vi "SP_OEE_2_test.vi"() -> ()   [LabVIEW 2017] (continued)
                          disable-tunnel: w4489 -> [w4505 w4508]
                          disable-tunnel: [w4504 w4508] -> w4488
                          disable-tunnel: [w4503 w4509] -> w4487
                          disable-tunnel: w4486 -> [w4502 _]
                          disable-tunnel: w4485 -> [w4501 _]
                          disable-tunnel: [w4500 _] -> w4484
                          disable-tunnel: [w4499 _] -> w4480
                          disable-tunnel: w4478 -> [w4498 _]
                          frame Disabled {
                            n825 = call "Stack_holderwise_total_bd_count_&_duration.vi"("Refnum in"=w4505, "BREAKDOWN_STK_HOLD_ID"=4, "condition"=w4498, "Form Date"=w4502, "To Date"=w4501, "error in (no error)"=w4506) -> ("Refnum out"=w4504:T2, "Count out"=w4500:string[], "appended array"=w4499:dbl[], "error out"=w4503:errorcluster)  [unwired: 6 in]
                          }
                          frame Enabled {
                          }
                        }
                        n826 = call "Insert_empty_element_with_zero.vi"("searched date"=w4484, "fixed date"=w4481) -> ("O/P"=w4483:string[])  [unwired: 9 in]
                        n827 = call "NUMERIC TO STRING.vi"("appended array"=w4480) -> ("Array"=w4479:string[])  [unwired: 4 in]
                        n828 = call "Insert_empty_element_with_zero.vi"("searched date"=w4479, "fixed date"=w4481) -> ("O/P"=w4482:string[])  [unwired: 9 in]
                      }
                      frame #5 {
                        n829 = disable-structure shown="Enabled" {
                          disable-tunnel: w4523 -> [w4541 w4544]
                          disable-tunnel: [w4540 w4544] -> w4522
                          disable-tunnel: w4521 -> [w4539 w4543]
                          disable-tunnel: [w4538 w4543] -> w4520
                          disable-tunnel: w4519 -> [w4537 _]
                          disable-tunnel: w4518 -> [w4536 _]
                          disable-tunnel: [w4535 _] -> w4517
                          disable-tunnel: [w4534 _] -> w4513
                          disable-tunnel: w4511 -> [w4533 _]
                          frame Disabled {
                            n830 = call "Stack_holderwise_total_bd_count_&_duration.vi"("Refnum in"=w4539, "BREAKDOWN_STK_HOLD_ID"=5, "condition"=w4533, "Form Date"=w4536, "To Date"=w4537, "error in (no error)"=w4541) -> ("Refnum out"=w4538:T2, "Count out"=w4535:string[], "appended array"=w4534:dbl[], "error out"=w4540:errorcluster)  [unwired: 6 in]
                          }
                          frame Enabled {
                          }
                        }
                        n831 = call "NUMERIC TO STRING.vi"("appended array"=w4513) -> ("Array"=w4512:string[])  [unwired: 4 in]
                        n832 = call "Insert_empty_element_with_zero.vi"("searched date"=w4517, "fixed date"=w4515) -> ("O/P"=w4516:string[])  [unwired: 9 in]
                        n833 = call "Insert_empty_element_with_zero.vi"("searched date"=w4512, "fixed date"=w4515) -> ("O/P"=w4514:string[])  [unwired: 9 in]
                      }
                      frame #6 {
                        n834 = call "String to numeric.vi"("Array"=w4555) -> ("Array 2"=w4554:dbl[])  [unwired: 4 in]
                        n835 = call "String to numeric.vi"("Array"=w4553) -> ("Array 2"=w4552:dbl[])  [unwired: 4 in]
                        n836 = call "String to numeric.vi"("Array"=w4551) -> ("Array 2"=w4550:dbl[])  [unwired: 4 in]
                        n837 = call "String to numeric.vi"("Array"=w4549) -> ("Array 2"=w4548:dbl[])  [unwired: 4 in]
                        n838 = call "String to numeric.vi"("Array"=w4547) -> ("Array 2"=w4546:dbl[])  [unwired: 4 in]
                        n839 = Decimal String To Number(string=w4560) -> (number=w4579:i32[])  [unwired: 2 in, 1 out]
                        n840 = Decimal String To Number(string=w4561) -> (number=w4580:i32[])  [unwired: 2 in, 1 out]
                        n841 = Decimal String To Number(string=w4562) -> (number=w4581:i32[])  [unwired: 2 in, 1 out]
                        n842 = Decimal String To Number(string=w4563) -> (number=w4582:i32[])  [unwired: 2 in, 1 out]
                        n843 = Decimal String To Number(string=w4564) -> (number=w4577:i32[])  [unwired: 2 in, 1 out]
                        n844 = Compound Arithmetic op=ADD(w4554, w4552, w4550, w4548, w4546) -> (w4557:dbl[])
                        n845 = Build Array(w4555) -> (w4576:string[][])
                        n846 = Build Array(w4553) -> (w4575:string[][])
                        n847 = Build Array(w4551) -> (w4574:string[][])
                        n848 = Build Array(w4549) -> (w4573:string[][])
                        n849 = Build Array(w4547) -> (w4572:string[][])
                        n850 = Number To Fractional String(number=w4557, precision (6)=i16 2) -> (F-format string=w4556:string[])  [unwired: 2 in]
                        n851 = Compound Arithmetic op=ADD(w4579, w4580, w4581, w4582, w4577) -> (w4583:i32[])
                        n852 = Transpose 2D Array(2D array=w4576) -> (transposed array=w4570:string[][])
                        n853 = Transpose 2D Array(2D array=w4575) -> (transposed array=w4569:string[][])
                        n854 = Transpose 2D Array(2D array=w4574) -> (transposed array=w4568:string[][])
                        n855 = Transpose 2D Array(2D array=w4573) -> (transposed array=w4567:string[][])
                        n856 = Transpose 2D Array(2D array=w4572) -> (transposed array=w4566:string[][])
                        n857 = Number To Decimal String(number=w4583) -> (decimal integer string=w4578:string[])  [unwired: 1 in]
                        n858 = Build Array(w4556) -> (w4559:string[][])
                        n859 = Transpose 2D Array(2D array=w4559) -> (transposed array=w4565:string[][])
                      }
                      frame #7 {
                        w4587 = string[] [""]
                        n860 = Insert Into Array(array=w4597, index (col)=1 ("disabled index (col)"), new element #1=w4587, new element #2=w4587, new element #3=w4588, new element #4=w4589, new element #5=w4587, new element #6=w4587, new element #7=w4587, new element #8=w4587, new element #9=w4587, new element #10=w4587, new element #11=w4590, new element #12=w4591) -> (w4593:string[][])  [unwired: 1 in]
                        n861 = call "flot graph for month n year.vi"("BD Date"=w4594, "error in (no error)"=w4596, "Count total"=w4590) -> ("error out"=w4595:errorcluster, "Run-Time Status"=w4592:cluster{"Array 2":timestamp[], dbl[]})  [unwired: 7 in]
                        n862 = local write "Run-Time Status"(w4592) -> ()
                        n863 = local write "Table"(w4593) -> ()
                      }
                    }
                  }
                  frame "all" {
                  }
                }
              }
              frame "Maintenance" {
                n864 = local read "Shift"() -> (w4599:string)
                n865 = case shown="\"1\"" w4599 {
                  selector: w4599 -> [_ w4972 w5351 w5730 _]
                  tunnel: w4604 -> [w4609 w4977 w5356 w5735 _]
                  tunnel: w4603 -> [w4608 w4976 w5355 w5734 _]
                  tunnel: w4602 -> [w4607 w4975 w5354 w5733 _]
                  tunnel: w4601 -> [w4606 w4974 w5353 w5732 _]
                  tunnel: w4600 -> [w4605 w4973 w5352 w5731 _]
                  frame "ALL", Default {
                    n866 = flat-sequence {
                      tunnel: w4609 -> [w4721]
                      tunnel: w4608 -> [w4719]
                      tunnel: [w4705] -> w4699
                      tunnel: [w4720] -> w4698
                      tunnel: w4607 -> [_]
                      tunnel: [w4724] -> w4697
                      tunnel: [w4704] -> w4696
                      tunnel: [w4703] -> w4695
                      tunnel: [w4701] -> w4694
                      tunnel: w4606 -> [w4704]
                      tunnel: w4605 -> [w4703]
                      tunnel: ["Where BREAKDOWN_DATE between '%s'and '%s' and BREAKDOWN_STK_HOLD_ID ='%d'  "] -> w4693
                      tunnel: [w4701] -> w4692
                      tunnel: w4699 -> [w4783]
                      tunnel: w4698 -> [w4785]
                      tunnel: w4697 -> [w4781]
                      tunnel: w4696 -> [w4780]
                      tunnel: w4695 -> [w4779]
                      tunnel: [w4782] -> w4691
                      tunnel: [w4784] -> w4690
                      tunnel: [w4781] -> w4689
                      tunnel: [w4771] -> w4688
                      tunnel: [w4777] -> w4687
                      tunnel: [w4780] -> w4686
                      tunnel: [w4779] -> w4685
                      tunnel: w4694 -> [w4776]
                      tunnel: [w4776] -> w4684
                      tunnel: w4693 -> [w4773]
                      tunnel: [w4773] -> w4683
                      tunnel: [w4772] -> w4682
                      tunnel: w4692 -> [w4772]
                      tunnel: w4691 -> [w4811]
                      tunnel: w4690 -> [w4809]
                      tunnel: w4689 -> [w4814]
                      tunnel: w4688 -> [w4813]
                      tunnel: w4687 -> [w4812]
                      tunnel: w4686 -> [w4807]
                      tunnel: w4685 -> [w4806]
                      tunnel: [w4814] -> w4681
                      tunnel: [w4813] -> w4680
                      tunnel: [w4812] -> w4679
                      tunnel: [w4810] -> w4678
                      tunnel: [w4804] -> w4677
                      tunnel: [w4803] -> w4676
                      tunnel: [w4808] -> w4675
                      tunnel: [w4807] -> w4674
                      tunnel: [w4806] -> w4673
                      tunnel: w4684 -> [w4802]
                      tunnel: [w4802] -> w4672
                      tunnel: w4683 -> [w4799]
                      tunnel: [w4799] -> w4671
                      tunnel: [w4798] -> w4670
                      tunnel: w4682 -> [w4798]
                      tunnel: w4681 -> [w4846]
                      tunnel: w4680 -> [w4845]
                      tunnel: w4679 -> [w4844]
                      tunnel: w4678 -> [w4841]
                      tunnel: w4677 -> [w4843]
                      tunnel: w4676 -> [w4842]
                      tunnel: w4675 -> [w4839]
                      tunnel: w4674 -> [w4837]
                      tunnel: w4673 -> [w4836]
                      tunnel: [w4846] -> w4669
                      tunnel: [w4845] -> w4668
                      tunnel: [w4844] -> w4667
                      tunnel: [w4843] -> w4666
                      tunnel: [w4842] -> w4665
                      tunnel: [w4840] -> w4664
                      tunnel: [w4834] -> w4663
                      tunnel: [w4833] -> w4662
                      tunnel: [w4838] -> w4661
                      tunnel: [w4837] -> w4660
                      tunnel: [w4836] -> w4659
                      tunnel: w4672 -> [w4832]
                      tunnel: [w4832] -> w4658
                      tunnel: w4671 -> [w4829]
                      tunnel: [w4829] -> w4657
                      tunnel: [w4828] -> w4656
                      tunnel: w4670 -> [w4828]
                      tunnel: w4669 -> [w4867]
                      tunnel: w4668 -> [w4866]
                      tunnel: w4667 -> [w4865]
                      tunnel: w4666 -> [w4864]
                      tunnel: w4665 -> [w4863]
                      tunnel: w4664 -> [w4860]
                      tunnel: w4663 -> [w4862]
                      tunnel: w4662 -> [w4861]
                      tunnel: w4661 -> [w4859]
                      tunnel: w4660 -> [w4856]
                      tunnel: w4659 -> [w4855]
                      tunnel: [w4867] -> w4655
                      tunnel: [w4866] -> w4654
                      tunnel: [w4865] -> w4653
                      tunnel: [w4864] -> w4652
                      tunnel: [w4863] -> w4651
                      tunnel: [w4862] -> w4650
                      tunnel: [w4861] -> w4649
                      tunnel: [w4858] -> w4648
                      tunnel: [w4857] -> w4647
                      tunnel: [w4853] -> w4646
                      tunnel: [w4852] -> w4645
                      tunnel: [w4856] -> w4644
                      tunnel: [w4855] -> w4643
                      tunnel: w4658 -> [w4851]
                      tunnel: [w4851] -> w4642
                      tunnel: w4657 -> [w4848]
                      tunnel: [w4848] -> w4641
                      tunnel: [w4847] -> w4640
                      tunnel: w4656 -> [w4847]
                      tunnel: w4655 -> [w4902]
                      tunnel: w4654 -> [w4901]
                      tunnel: w4653 -> [w4900]
                      tunnel: w4652 -> [w4899]
                      tunnel: w4651 -> [w4898]
                      tunnel: w4650 -> [w4897]
                      tunnel: w4649 -> [w4896]
                      tunnel: w4648 -> [w4891]
                      tunnel: w4647 -> [w4893]
                      tunnel: w4646 -> [w4895]
                      tunnel: w4645 -> [w4894]
                      tunnel: w4644 -> [w4888]
                      tunnel: w4643 -> [w4889]
                      tunnel: [w4902] -> w4639
                      tunnel: [w4901] -> w4638
                      tunnel: [w4900] -> w4637
                      tunnel: [w4899] -> w4636
                      tunnel: [w4898] -> w4635
                      tunnel: [w4897] -> w4634
                      tunnel: [w4896] -> w4633
                      tunnel: [w4895] -> w4632
                      tunnel: [w4894] -> w4631
                      tunnel: [w4892] -> w4630
                      tunnel: [w4890] -> w4629
                      tunnel: [w4886] -> w4628
                      tunnel: [w4884] -> w4627
                      tunnel: w4642 -> [w4885]
                      tunnel: w4641 -> [w4881]
                      tunnel: [w4880] -> w4626
                      tunnel: w4640 -> [w4880]
                      tunnel: w4639 -> [w4941]
                      tunnel: w4638 -> [w4934]
                      tunnel: w4637 -> [w4925]
                      tunnel: w4636 -> [w4933]
                      tunnel: w4635 -> [w4923]
                      tunnel: w4634 -> [w4932]
                      tunnel: w4633 -> [w4921]
                      tunnel: w4632 -> [w4931]
                      tunnel: w4631 -> [w4919]
                      tunnel: w4630 -> [w4955]
                      tunnel: w4629 -> [w4954]
                      tunnel: w4628 -> [w4930]
                      tunnel: w4627 -> [w4917]
                      tunnel: [w4955] -> w4625
                      tunnel: [w4954] -> w4624
                      tunnel: [w4948] -> w4623
                      tunnel: [w4941] -> w4622
                      tunnel: [w4940] -> w4621
                      tunnel: [w4939] -> w4620
                      tunnel: [w4938] -> w4619
                      tunnel: [w4937] -> w4618
                      tunnel: [w4936] -> w4617
                      tunnel: [w4935] -> w4616
                      tunnel: [w4934] -> w4615
                      tunnel: [w4933] -> w4614
                      tunnel: [w4932] -> w4613
                      tunnel: [w4931] -> w4612
                      tunnel: [w4930] -> w4611
                      tunnel: [w4915] -> w4610
                      tunnel: w4626 -> [w4915]
                      tunnel: [w4968] -> _
                      tunnel: [w4964] -> _
                      tunnel: w4625 -> [w4965]
                      tunnel: w4624 -> [w4968]
                      tunnel: w4623 -> [w4959]
                      tunnel: w4622 -> [w4966]
                      tunnel: w4621 -> [_]
                      tunnel: w4620 -> [_]
                      tunnel: w4619 -> [w4956]
                      tunnel: w4618 -> [_]
                      tunnel: w4617 -> [_]
                      tunnel: w4616 -> [w4960]
                      tunnel: w4615 -> [_]
                      tunnel: w4614 -> [_]
                      tunnel: w4613 -> [w4957]
                      tunnel: w4612 -> [_]
                      tunnel: w4611 -> [_]
                      tunnel: w4610 -> [w4963]
                      frame #0 {
                        w4712 = "%Y-%m-%d" ("time format string (%c)")
                        n867 = property on="Table" class="Tbl (strict)"("Visible"=TRUE) -> ()  [unwired: 2 in, 2 out]
                        n868 = Format Date/Time String(time format string (%c)=w4712, seconds (now)=w4704) -> (date/time string=w4713:string)  [unwired: 1 in]
                        n869 = Format Date/Time String(time format string (%c)=w4712, seconds (now)=w4703) -> (date/time string=w4711:string)  [unwired: 1 in]
                        n870 = Format Into String(format string="Where BREAKDOWN_DATE between '%s' and '%s' ", w4713, w4711) -> (resulting string=w4710:string)  [unwired: 2 in, 1 out]
                        n871 = call <vilib>:"DB Tools Select Data.vi"("condition"=w4710, "error in (no error)"=w4719, "columns"=string[] ["BREAKDOWN_DATE"], "table"="STATION_1_LOG_HISTORY", "connection reference"=w4721) -> ("error out"=w4706:errorcluster, "data"=w4709:variant[][], "connection reference out"=w4720:T2)  [unwired: 1 in]
                        n872 = property on="Table 2" class="Tbl (strict)"("Visible"=FALSE) -> ()  [unwired: 2 in, 2 out]
                        n873 = xnode "Database Variant To Data"("database variant"=w4709, "error in (no error)"=w4706, "type"=string[][] [] ("Elements Found")) -> ("data"=w4707:string[][], "error out"=w4705:errorcluster)
                        n874 = Index Array(array=w4707, index (col)=0 ("disabled index (col)")) -> (element=w4715:string[])  [unwired: 1 in]
                        n875 = call "Search_1d_array_element.vi"("Count in"=string[] [] ("Elements Found"), "BD Date"=w4715, "Elements Found in"=string[] [] ("Elements Found")) -> ("Elements Found out"=w4701:string[])  [unwired: 4 in, 2 out]
                        n876 = Build Array(w4701) -> (w4725:string[][])
                        n877 = Transpose 2D Array(2D array=w4725) -> (transposed array=w4724:string[][])
                      }
                      frame #1 {
                        n878 = disable-structure shown="Enabled" {
                          disable-tunnel: w4785 -> [w4795 w4796]
                          disable-tunnel: [w4794 w4796] -> w4784
                          disable-tunnel: w4783 -> [w4793 w4797]
                          disable-tunnel: [w4792 w4797] -> w4782
                          disable-tunnel: w4780 -> [w4790 _]
                          disable-tunnel: w4779 -> [w4789 _]
                          disable-tunnel: [w4788 _] -> w4778
                          disable-tunnel: [w4787 _] -> w4775
                          disable-tunnel: w4773 -> [w4786 _]
                          frame Disabled {
                            n879 = call "Stack_holderwise_total_bd_count_&_duration.vi"("Refnum in"=w4795, "BREAKDOWN_STK_HOLD_ID"=1, "condition"=w4786, "Form Date"=w4790, "To Date"=w4789, "error in (no error)"=w4793) -> ("Refnum out"=w4794:T2, "Count out"=w4788:string[], "appended array"=w4787:dbl[], "error out"=w4792:errorcluster)  [unwired: 6 in]
                          }
                          frame Enabled {
                          }
                        }
                        n880 = call "NUMERIC TO STRING.vi"("appended array"=w4775) -> ("Array"=w4774:string[])  [unwired: 4 in]
                        n881 = call "Insert_empty_element_with_zero.vi"("searched date"=w4778, "fixed date"=w4776) -> ("O/P"=w4771:string[])  [unwired: 9 in]
                        n882 = call "Insert_empty_element_with_zero.vi"("searched date"=w4774, "fixed date"=w4776) -> ("O/P"=w4777:string[])  [unwired: 9 in]
                      }
                      frame #2 {
                        n883 = disable-structure shown="Enabled" {
                          disable-tunnel: w4811 -> [w4824 w4826]
                          disable-tunnel: [w4823 w4826] -> w4810
                          disable-tunnel: w4809 -> [w4822 w4825]
                          disable-tunnel: [w4821 w4825] -> w4808
                          disable-tunnel: w4807 -> [w4820 _]
                          disable-tunnel: w4806 -> [w4819 _]
                          disable-tunnel: [w4818 _] -> w4805
                          disable-tunnel: [w4817 _] -> w4801
                          disable-tunnel: w4799 -> [w4816 _]
                          frame Disabled {
                            n884 = call "Stack_holderwise_total_bd_count_&_duration.vi"("Refnum in"=w4822, "BREAKDOWN_STK_HOLD_ID"=2, "condition"=w4816, "Form Date"=w4820, "To Date"=w4819, "error in (no error)"=w4824) -> ("Refnum out"=w4821:T2, "Count out"=w4818:string[], "appended array"=w4817:dbl[], "error out"=w4823:errorcluster)  [unwired: 6 in]
                          }
                          frame Enabled {
                          }
                        }
                        n885 = call "Insert_empty_element_with_zero.vi"("searched date"=w4805, "fixed date"=w4802) -> ("O/P"=w4804:string[])  [unwired: 9 in]
                        n886 = call "NUMERIC TO STRING.vi"("appended array"=w4801) -> ("Array"=w4800:string[])  [unwired: 4 in]
                        n887 = call "Insert_empty_element_with_zero.vi"("searched date"=w4800, "fixed date"=w4802) -> ("O/P"=w4803:string[])  [unwired: 9 in]
                      }
                      frame #3 {
                        n888 = call "Stack_holderwise_total_bd_count_&_duration.vi"("Refnum in"=w4839, "BREAKDOWN_STK_HOLD_ID"=3, "condition"=w4829, "Form Date"=w4837, "To Date"=w4836, "error in (no error)"=w4841) -> ("Refnum out"=w4838:T2, "Count out"=w4835:string[], "appended array"=w4831:dbl[], "error out"=w4840:errorcluster)  [unwired: 6 in]
                        n889 = call "Insert_empty_element_with_zero.vi"("searched date"=w4835, "fixed date"=w4832) -> ("O/P"=w4834:string[])  [unwired: 9 in]
                        n890 = call "NUMERIC TO STRING.vi"("appended array"=w4831) -> ("Array"=w4830:string[])  [unwired: 4 in]
                        n891 = call "Insert_empty_element_with_zero.vi"("searched date"=w4830, "fixed date"=w4832) -> ("O/P"=w4833:string[])  [unwired: 9 in]
                      }
                      frame #4 {
                        n892 = disable-structure shown="Enabled" {
                          disable-tunnel: w4860 -> [w4876 w4879]
                          disable-tunnel: w4859 -> [w4875 w4878]
                          disable-tunnel: [w4874 w4878] -> w4858
                          disable-tunnel: [w4873 w4879] -> w4857
                          disable-tunnel: w4856 -> [w4872 _]
                          disable-tunnel: w4855 -> [w4871 _]
                          disable-tunnel: [w4870 _] -> w4854
                          disable-tunnel: [w4869 _] -> w4850
                          disable-tunnel: w4848 -> [w4868 _]
                          frame Disabled {
                            n893 = call "Stack_holderwise_total_bd_count_&_duration.vi"("Refnum in"=w4875, "BREAKDOWN_STK_HOLD_ID"=4, "condition"=w4868, "Form Date"=w4872, "To Date"=w4871, "error in (no error)"=w4876) -> ("Refnum out"=w4874:T2, "Count out"=w4870:string[], "appended array"=w4869:dbl[], "error out"=w4873:errorcluster)  [unwired: 6 in]
                          }
                          frame Enabled {
                          }
                        }
                        n894 = call "Insert_empty_element_with_zero.vi"("searched date"=w4854, "fixed date"=w4851) -> ("O/P"=w4853:string[])  [unwired: 9 in]
                        n895 = call "NUMERIC TO STRING.vi"("appended array"=w4850) -> ("Array"=w4849:string[])  [unwired: 4 in]
                        n896 = call "Insert_empty_element_with_zero.vi"("searched date"=w4849, "fixed date"=w4851) -> ("O/P"=w4852:string[])  [unwired: 9 in]
                      }
                      frame #5 {
                        n897 = disable-structure shown="Enabled" {
                          disable-tunnel: w4893 -> [w4911 w4914]
                          disable-tunnel: [w4910 w4914] -> w4892
                          disable-tunnel: w4891 -> [w4909 w4913]
                          disable-tunnel: [w4908 w4913] -> w4890
                          disable-tunnel: w4889 -> [w4907 _]
                          disable-tunnel: w4888 -> [w4906 _]
                          disable-tunnel: [w4905 _] -> w4887
                          disable-tunnel: [w4904 _] -> w4883
                          disable-tunnel: w4881 -> [w4903 _]
                          frame Disabled {
                            n898 = call "Stack_holderwise_total_bd_count_&_duration.vi"("Refnum in"=w4909, "BREAKDOWN_STK_HOLD_ID"=5, "condition"=w4903, "Form Date"=w4906, "To Date"=w4907, "error in (no error)"=w4911) -> ("Refnum out"=w4908:T2, "Count out"=w4905:string[], "appended array"=w4904:dbl[], "error out"=w4910:errorcluster)  [unwired: 6 in]
                          }
                          frame Enabled {
                          }
                        }
                        n899 = call "NUMERIC TO STRING.vi"("appended array"=w4883) -> ("Array"=w4882:string[])  [unwired: 4 in]
                        n900 = call "Insert_empty_element_with_zero.vi"("searched date"=w4887, "fixed date"=w4885) -> ("O/P"=w4886:string[])  [unwired: 9 in]
                        n901 = call "Insert_empty_element_with_zero.vi"("searched date"=w4882, "fixed date"=w4885) -> ("O/P"=w4884:string[])  [unwired: 9 in]
                      }
                      frame #6 {
                        n902 = call "String to numeric.vi"("Array"=w4925) -> ("Array 2"=w4924:dbl[])  [unwired: 4 in]
                        n903 = call "String to numeric.vi"("Array"=w4923) -> ("Array 2"=w4922:dbl[])  [unwired: 4 in]
                        n904 = call "String to numeric.vi"("Array"=w4921) -> ("Array 2"=w4920:dbl[])  [unwired: 4 in]
                        n905 = call "String to numeric.vi"("Array"=w4919) -> ("Array 2"=w4918:dbl[])  [unwired: 4 in]
                        n906 = call "String to numeric.vi"("Array"=w4917) -> ("Array 2"=w4916:dbl[])  [unwired: 4 in]
                        n907 = Decimal String To Number(string=w4930) -> (number=w4949:i32[])  [unwired: 2 in, 1 out]
                        n908 = Decimal String To Number(string=w4931) -> (number=w4950:i32[])  [unwired: 2 in, 1 out]
                        n909 = Decimal String To Number(string=w4932) -> (number=w4951:i32[])  [unwired: 2 in, 1 out]
                        n910 = Decimal String To Number(string=w4933) -> (number=w4952:i32[])  [unwired: 2 in, 1 out]
                        n911 = Decimal String To Number(string=w4934) -> (number=w4947:i32[])  [unwired: 2 in, 1 out]
                        n912 = Compound Arithmetic op=ADD(w4924, w4922, w4920, w4918, w4916) -> (w4927:dbl[])
                        n913 = Build Array(w4925) -> (w4946:string[][])
                        n914 = Build Array(w4923) -> (w4945:string[][])
                        n915 = Build Array(w4921) -> (w4944:string[][])
                        n916 = Build Array(w4919) -> (w4943:string[][])
                        n917 = Build Array(w4917) -> (w4942:string[][])
                        n918 = Number To Fractional String(number=w4927, precision (6)=i16 2) -> (F-format string=w4926:string[])  [unwired: 2 in]
                        n919 = Compound Arithmetic op=ADD(w4949, w4950, w4951, w4952, w4947) -> (w4953:i32[])
                        n920 = Transpose 2D Array(2D array=w4946) -> (transposed array=w4940:string[][])
                        n921 = Transpose 2D Array(2D array=w4945) -> (transposed array=w4939:string[][])
                        n922 = Transpose 2D Array(2D array=w4944) -> (transposed array=w4938:string[][])
                        n923 = Transpose 2D Array(2D array=w4943) -> (transposed array=w4937:string[][])
                        n924 = Transpose 2D Array(2D array=w4942) -> (transposed array=w4936:string[][])
                        n925 = Number To Decimal String(number=w4953) -> (decimal integer string=w4948:string[])  [unwired: 1 in]
                        n926 = Build Array(w4926) -> (w4929:string[][])
                        n927 = Transpose 2D Array(2D array=w4929) -> (transposed array=w4935:string[][])
                      }
                      frame #7 {
                        w4958 = string[] [""]
                        n928 = Insert Into Array(array=w4966, index (col)=1 ("disabled index (col)"), new element #1=w4958, new element #2=w4958, new element #3=w4958, new element #4=w4958, new element #5=w4957, new element #6=w4956, new element #7=w4958, new element #8=w4958, new element #9=w4958, new element #10=w4958, new element #11=w4959, new element #12=w4960) -> (w4962:string[][])  [unwired: 1 in]
                        n929 = call "flot graph for month n year.vi"("BD Date"=w4963, "error in (no error)"=w4965, "Count total"=w4959) -> ("error out"=w4964:errorcluster, "Run-Time Status"=w4961:cluster{"Array 2":timestamp[], dbl[]})  [unwired: 7 in]
                        n930 = local write "Run-Time Status"(w4961) -> ()
                        n931 = local write "Table"(w4962) -> ()
                      }
                    }
                  }
                  frame "1" {
                    n932 = flat-sequence {
                      tunnel: w4977 -> [w5091]
                      tunnel: w4976 -> [w5089]
                      tunnel: [w5075] -> w5067
                      tunnel: [w5090] -> w5066
                      tunnel: w4975 -> [_]
                      tunnel: [w5094] -> w5065
                      tunnel: [w5074] -> w5064
                      tunnel: [w5073] -> w5063
                      tunnel: [w5072] -> w5062
                      tunnel: w4974 -> [w5074]
                      tunnel: w4973 -> [w5073]
                      tunnel: ["Where BREAKDOWN_DATE between '%s'and '%s' and BREAKDOWN_STK_HOLD_ID ='%d' and  SHIFT_ID = '%d' "] -> w5061
                      tunnel: [w5072] -> w5060
                      tunnel: w4972 -> [w5068]
                      tunnel: [w5068] -> w4971
                      tunnel: w5067 -> [w5155]
                      tunnel: w5066 -> [w5157]
                      tunnel: w5065 -> [w5153]
                      tunnel: w5064 -> [w5152]
                      tunnel: w5063 -> [w5151]
                      tunnel: [w5154] -> w5059
                      tunnel: [w5156] -> w5058
                      tunnel: [w5153] -> w5057
                      tunnel: [w5143] -> w5056
                      tunnel: [w5149] -> w5055
                      tunnel: [w5152] -> w5054
                      tunnel: [w5151] -> w5053
                      tunnel: w5062 -> [w5148]
                      tunnel: [w5148] -> w5052
                      tunnel: w5061 -> [w5145]
                      tunnel: [w5145] -> w5051
                      tunnel: [w5144] -> w5050
                      tunnel: w5060 -> [w5144]
                      tunnel: w4971 -> [w5142]
                      tunnel: [w5141] -> w4970
                      tunnel: w5059 -> [w5187]
                      tunnel: w5058 -> [w5185]
                      tunnel: w5057 -> [w5190]
                      tunnel: w5056 -> [w5189]
                      tunnel: w5055 -> [w5188]
                      tunnel: w5054 -> [w5183]
                      tunnel: w5053 -> [w5182]
                      tunnel: [w5190] -> w5049
                      tunnel: [w5189] -> w5048
                      tunnel: [w5188] -> w5047
                      tunnel: [w5186] -> w5046
                      tunnel: [w5180] -> w5045
                      tunnel: [w5179] -> w5044
                      tunnel: [w5184] -> w5043
                      tunnel: [w5183] -> w5042
                      tunnel: [w5182] -> w5041
                      tunnel: w5052 -> [w5178]
                      tunnel: [w5178] -> w5040
                      tunnel: w5051 -> [w5175]
                      tunnel: [w5175] -> w5039
                      tunnel: [w5174] -> w5038
                      tunnel: w5050 -> [w5174]
                      tunnel: w4970 -> [w5173]
                      tunnel: [w5172] -> w4969
                      tunnel: w5049 -> [w5225]
                      tunnel: w5048 -> [w5224]
                      tunnel: w5047 -> [w5223]
                      tunnel: w5046 -> [w5220]
                      tunnel: w5045 -> [w5222]
                      tunnel: w5044 -> [w5221]
                      tunnel: w5043 -> [w5218]
                      tunnel: w5042 -> [w5216]
                      tunnel: w5041 -> [w5215]
                      tunnel: [w5225] -> w5037
                      tunnel: [w5224] -> w5036
                      tunnel: [w5223] -> w5035
                      tunnel: [w5222] -> w5034
                      tunnel: [w5221] -> w5033
                      tunnel: [w5219] -> w5032
                      tunnel: [w5213] -> w5031
                      tunnel: [w5212] -> w5030
                      tunnel: [w5217] -> w5029
                      tunnel: [w5216] -> w5028
                      tunnel: [w5215] -> w5027
                      tunnel: w5040 -> [w5211]
                      tunnel: [w5211] -> w5026
                      tunnel: w5039 -> [w5208]
                      tunnel: [w5208] -> w5025
                      tunnel: [w5207] -> w5024
                      tunnel: w5038 -> [w5207]
                      tunnel: w4969 -> [w5205]
                      tunnel: w5037 -> [w5246]
                      tunnel: w5036 -> [w5245]
                      tunnel: w5035 -> [w5244]
                      tunnel: w5034 -> [w5243]
                      tunnel: w5033 -> [w5242]
                      tunnel: w5032 -> [w5239]
                      tunnel: w5031 -> [w5241]
                      tunnel: w5030 -> [w5240]
                      tunnel: w5029 -> [w5238]
                      tunnel: w5028 -> [w5235]
                      tunnel: w5027 -> [w5234]
                      tunnel: [w5246] -> w5023
                      tunnel: [w5245] -> w5022
                      tunnel: [w5244] -> w5021
                      tunnel: [w5243] -> w5020
                      tunnel: [w5242] -> w5019
                      tunnel: [w5241] -> w5018
                      tunnel: [w5240] -> w5017
                      tunnel: [w5237] -> w5016
                      tunnel: [w5236] -> w5015
                      tunnel: [w5232] -> w5014
                      tunnel: [w5231] -> w5013
                      tunnel: [w5235] -> w5012
                      tunnel: [w5234] -> w5011
                      tunnel: w5026 -> [w5230]
                      tunnel: [w5230] -> w5010
                      tunnel: w5025 -> [w5227]
                      tunnel: [w5227] -> w5009
                      tunnel: [w5226] -> w5008
                      tunnel: w5024 -> [w5226]
                      tunnel: w5023 -> [w5281]
                      tunnel: w5022 -> [w5280]
                      tunnel: w5021 -> [w5279]
                      tunnel: w5020 -> [w5278]
                      tunnel: w5019 -> [w5277]
                      tunnel: w5018 -> [w5276]
                      tunnel: w5017 -> [w5275]
                      tunnel: w5016 -> [w5270]
                      tunnel: w5015 -> [w5272]
                      tunnel: w5014 -> [w5274]
                      tunnel: w5013 -> [w5273]
                      tunnel: w5012 -> [w5267]
                      tunnel: w5011 -> [w5268]
                      tunnel: [w5281] -> w5007
                      tunnel: [w5280] -> w5006
                      tunnel: [w5279] -> w5005
                      tunnel: [w5278] -> w5004
                      tunnel: [w5277] -> w5003
                      tunnel: [w5276] -> w5002
                      tunnel: [w5275] -> w5001
                      tunnel: [w5274] -> w5000
                      tunnel: [w5273] -> w4999
                      tunnel: [w5271] -> w4998
                      tunnel: [w5269] -> w4997
                      tunnel: [w5265] -> w4996
                      tunnel: [w5263] -> w4995
                      tunnel: w5010 -> [w5264]
                      tunnel: w5009 -> [w5260]
                      tunnel: [w5259] -> w4994
                      tunnel: w5008 -> [w5259]
                      tunnel: w5007 -> [w5320]
                      tunnel: w5006 -> [w5313]
                      tunnel: w5005 -> [w5304]
                      tunnel: w5004 -> [w5312]
                      tunnel: w5003 -> [w5302]
                      tunnel: w5002 -> [w5311]
                      tunnel: w5001 -> [w5300]
                      tunnel: w5000 -> [w5310]
                      tunnel: w4999 -> [w5298]
                      tunnel: w4998 -> [w5334]
                      tunnel: w4997 -> [w5333]
                      tunnel: w4996 -> [w5309]
                      tunnel: w4995 -> [w5296]
                      tunnel: [w5334] -> w4993
                      tunnel: [w5333] -> w4992
                      tunnel: [w5327] -> w4991
                      tunnel: [w5320] -> w4990
                      tunnel: [w5319] -> w4989
                      tunnel: [w5318] -> w4988
                      tunnel: [w5317] -> w4987
                      tunnel: [w5316] -> w4986
                      tunnel: [w5315] -> w4985
                      tunnel: [w5314] -> w4984
                      tunnel: [w5313] -> w4983
                      tunnel: [w5312] -> w4982
                      tunnel: [w5311] -> w4981
                      tunnel: [w5310] -> w4980
                      tunnel: [w5309] -> w4979
                      tunnel: [w5294] -> w4978
                      tunnel: w4994 -> [w5294]
                      tunnel: [w5347] -> _
                      tunnel: [w5343] -> _
                      tunnel: w4993 -> [w5344]
                      tunnel: w4992 -> [w5347]
                      tunnel: w4991 -> [w5338]
                      tunnel: w4990 -> [w5345]
                      tunnel: w4989 -> [_]
                      tunnel: w4988 -> [_]
                      tunnel: w4987 -> [w5337]
                      tunnel: w4986 -> [_]
                      tunnel: w4985 -> [_]
                      tunnel: w4984 -> [w5339]
                      tunnel: w4983 -> [_]
                      tunnel: w4982 -> [_]
                      tunnel: w4981 -> [w5335]
                      tunnel: w4980 -> [_]
                      tunnel: w4979 -> [_]
                      tunnel: w4978 -> [w5342]
                      frame #0 {
                        w5082 = "%Y-%m-%d" ("time format string (%c)")
                        n933 = Decimal String To Number(string=w5068) -> (number=w5069:i32)  [unwired: 2 in, 1 out]
                        n934 = property on="Table" class="Tbl (strict)"("Visible"=TRUE) -> ()  [unwired: 2 in, 2 out]
                        n935 = Format Date/Time String(time format string (%c)=w5082, seconds (now)=w5074) -> (date/time string=w5083:string)  [unwired: 1 in]
                        n936 = Format Date/Time String(time format string (%c)=w5082, seconds (now)=w5073) -> (date/time string=w5081:string)  [unwired: 1 in]
                        n937 = Format Into String(format string="Where BREAKDOWN_DATE between '%s' and '%s' and  SHIFT_ID = '%d'  ", w5083, w5081, w5069) -> (resulting string=w5080:string)  [unwired: 2 in, 1 out]
                        n938 = call <vilib>:"DB Tools Select Data.vi"("condition"=w5080, "error in (no error)"=w5089, "columns"=string[] ["BREAKDOWN_DATE"], "table"="STATION_1_LOG_HISTORY", "connection reference"=w5091) -> ("error out"=w5076:errorcluster, "data"=w5079:variant[][], "connection reference out"=w5090:T2)  [unwired: 1 in]
                        n939 = property on="Table 2" class="Tbl (strict)"("Visible"=FALSE) -> ()  [unwired: 2 in, 2 out]
                        n940 = xnode "Database Variant To Data"("database variant"=w5079, "error in (no error)"=w5076, "type"=string[][] [] ("Elements Found")) -> ("data"=w5077:string[][], "error out"=w5075:errorcluster)
                        n941 = Index Array(array=w5077, index (col)=0 ("disabled index (col)")) -> (element=w5085:string[])  [unwired: 1 in]
                        n942 = call "Search_1d_array_element.vi"("Count in"=string[] [] ("Elements Found"), "BD Date"=w5085, "Elements Found in"=string[] [] ("Elements Found")) -> ("Elements Found out"=w5072:string[])  [unwired: 4 in, 2 out]
                        n943 = Build Array(w5072) -> (w5095:string[][])
                        n944 = Transpose 2D Array(2D array=w5095) -> (transposed array=w5094:string[][])
                      }
                      frame #1 {
                        n945 = disable-structure shown="Enabled" {
                          disable-tunnel: w5157 -> [w5168 w5170]
                          disable-tunnel: [w5167 w5170] -> w5156
                          disable-tunnel: w5155 -> [w5166 w5171]
                          disable-tunnel: [w5165 w5171] -> w5154
                          disable-tunnel: w5152 -> [w5163 _]
                          disable-tunnel: w5151 -> [w5162 _]
                          disable-tunnel: [w5161 _] -> w5150
                          disable-tunnel: [w5160 _] -> w5147
                          disable-tunnel: w5145 -> [w5159 _]
                          disable-tunnel: w5142 -> [w5158 w5169]
                          disable-tunnel: [_ w5169] -> w5141
                          frame Disabled {
                            n946 = call "Stack_holderwise_total_bd_count_&_duration_2.vi"("Refnum in"=w5168, "BREAKDOWN_STK_HOLD_ID"=1, "condition"=w5159, "Form Date"=w5163, "To Date"=w5162, "error in (no error)"=w5166, "Shift"=w5158) -> ("Refnum out"=w5167:T2, "Count out"=w5161:string[], "appended array"=w5160:dbl[], "error out"=w5165:errorcluster)  [unwired: 5 in]
                          }
                          frame Enabled {
                          }
                        }
                        n947 = call "NUMERIC TO STRING.vi"("appended array"=w5147) -> ("Array"=w5146:string[])  [unwired: 4 in]
                        n948 = call "Insert_empty_element_with_zero.vi"("searched date"=w5150, "fixed date"=w5148) -> ("O/P"=w5143:string[])  [unwired: 9 in]
                        n949 = call "Insert_empty_element_with_zero.vi"("searched date"=w5146, "fixed date"=w5148) -> ("O/P"=w5149:string[])  [unwired: 9 in]
                      }
                      frame #2 {
                        n950 = disable-structure shown="Enabled" {
                          disable-tunnel: w5187 -> [w5201 w5203]
                          disable-tunnel: [w5200 w5203] -> w5186
                          disable-tunnel: w5185 -> [w5199 w5204]
                          disable-tunnel: [w5198 w5204] -> w5184
                          disable-tunnel: w5183 -> [w5197 _]
                          disable-tunnel: w5182 -> [w5196 _]
                          disable-tunnel: [w5195 _] -> w5181
                          disable-tunnel: [w5194 _] -> w5177
                          disable-tunnel: w5175 -> [w5193 _]
                          disable-tunnel: w5173 -> [w5191 w5202]
                          disable-tunnel: [_ w5202] -> w5172
                          frame Disabled {
                            n951 = call "Stack_holderwise_total_bd_count_&_duration_2.vi"("Refnum in"=w5199, "BREAKDOWN_STK_HOLD_ID"=2, "condition"=w5193, "Form Date"=w5197, "To Date"=w5196, "error in (no error)"=w5201, "Shift"=w5191) -> ("Refnum out"=w5198:T2, "Count out"=w5195:string[], "appended array"=w5194:dbl[], "error out"=w5200:errorcluster)  [unwired: 5 in]
                          }
                          frame Enabled {
                          }
                        }
                        n952 = call "Insert_empty_element_with_zero.vi"("searched date"=w5181, "fixed date"=w5178) -> ("O/P"=w5180:string[])  [unwired: 9 in]
                        n953 = call "NUMERIC TO STRING.vi"("appended array"=w5177) -> ("Array"=w5176:string[])  [unwired: 4 in]
                        n954 = call "Insert_empty_element_with_zero.vi"("searched date"=w5176, "fixed date"=w5178) -> ("O/P"=w5179:string[])  [unwired: 9 in]
                      }
                      frame #3 {
                        n955 = call "Stack_holderwise_total_bd_count_&_duration_2.vi"("Refnum in"=w5218, "BREAKDOWN_STK_HOLD_ID"=3, "condition"=w5208, "Form Date"=w5216, "To Date"=w5215, "error in (no error)"=w5220, "Shift"=w5205) -> ("Refnum out"=w5217:T2, "Count out"=w5214:string[], "appended array"=w5210:dbl[], "error out"=w5219:errorcluster)  [unwired: 5 in]
                        n956 = call "Insert_empty_element_with_zero.vi"("searched date"=w5214, "fixed date"=w5211) -> ("O/P"=w5213:string[])  [unwired: 9 in]
                        n957 = call "NUMERIC TO STRING.vi"("appended array"=w5210) -> ("Array"=w5209:string[])  [unwired: 4 in]
                        n958 = call "Insert_empty_element_with_zero.vi"("searched date"=w5209, "fixed date"=w5211) -> ("O/P"=w5212:string[])  [unwired: 9 in]
                      }
                      frame #4 {
                        n959 = disable-structure shown="Enabled" {
                          disable-tunnel: w5239 -> [w5255 w5258]
                          disable-tunnel: w5238 -> [w5254 w5257]
                          disable-tunnel: [w5253 w5257] -> w5237
                          disable-tunnel: [w5252 w5258] -> w5236
                          disable-tunnel: w5235 -> [w5251 _]
                          disable-tunnel: w5234 -> [w5250 _]
                          disable-tunnel: [w5249 _] -> w5233
                          disable-tunnel: [w5248 _] -> w5229
                          disable-tunnel: w5227 -> [w5247 _]
                          frame Disabled {
                            n960 = call "Stack_holderwise_total_bd_count_&_duration.vi"("Refnum in"=w5254, "BREAKDOWN_STK_HOLD_ID"=4, "condition"=w5247, "Form Date"=w5251, "To Date"=w5250, "error in (no error)"=w5255) -> ("Refnum out"=w5253:T2, "Count out"=w5249:string[], "appended array"=w5248:dbl[], "error out"=w5252:errorcluster)  [unwired: 6 in]
                          }
                          frame Enabled {
                          }
                        }
                        n961 = call "Insert_empty_element_with_zero.vi"("searched date"=w5233, "fixed date"=w5230) -> ("O/P"=w5232:string[])  [unwired: 9 in]
                        n962 = call "NUMERIC TO STRING.vi"("appended array"=w5229) -> ("Array"=w5228:string[])  [unwired: 4 in]
                        n963 = call "Insert_empty_element_with_zero.vi"("searched date"=w5228, "fixed date"=w5230) -> ("O/P"=w5231:string[])  [unwired: 9 in]
                      }
                      frame #5 {
                        n964 = disable-structure shown="Enabled" {
                          disable-tunnel: w5272 -> [w5290 w5293]
                          disable-tunnel: [w5289 w5293] -> w5271
                          disable-tunnel: w5270 -> [w5288 w5292]
                          disable-tunnel: [w5287 w5292] -> w5269
                          disable-tunnel: w5268 -> [w5286 _]
                          disable-tunnel: w5267 -> [w5285 _]
                          disable-tunnel: [w5284 _] -> w5266
                          disable-tunnel: [w5283 _] -> w5262
                          disable-tunnel: w5260 -> [w5282 _]
                          frame Disabled {
                            n965 = call "Stack_holderwise_total_bd_count_&_duration.vi"("Refnum in"=w5288, "BREAKDOWN_STK_HOLD_ID"=5, "condition"=w5282, "Form Date"=w5285, "To Date"=w5286, "error in (no error)"=w5290) -> ("Refnum out"=w5287:T2, "Count out"=w5284:string[], "appended array"=w5283:dbl[], "error out"=w5289:errorcluster)  [unwired: 6 in]
                          }
                          frame Enabled {
                          }
                        }
                        n966 = call "NUMERIC TO STRING.vi"("appended array"=w5262) -> ("Array"=w5261:string[])  [unwired: 4 in]
                        n967 = call "Insert_empty_element_with_zero.vi"("searched date"=w5266, "fixed date"=w5264) -> ("O/P"=w5265:string[])  [unwired: 9 in]
                        n968 = call "Insert_empty_element_with_zero.vi"("searched date"=w5261, "fixed date"=w5264) -> ("O/P"=w5263:string[])  [unwired: 9 in]
                      }
                      frame #6 {
                        n969 = call "String to numeric.vi"("Array"=w5304) -> ("Array 2"=w5303:dbl[])  [unwired: 4 in]
                        n970 = call "String to numeric.vi"("Array"=w5302) -> ("Array 2"=w5301:dbl[])  [unwired: 4 in]
                        n971 = call "String to numeric.vi"("Array"=w5300) -> ("Array 2"=w5299:dbl[])  [unwired: 4 in]
                        n972 = call "String to numeric.vi"("Array"=w5298) -> ("Array 2"=w5297:dbl[])  [unwired: 4 in]
                        n973 = call "String to numeric.vi"("Array"=w5296) -> ("Array 2"=w5295:dbl[])  [unwired: 4 in]
                        n974 = Decimal String To Number(string=w5309) -> (number=w5328:i32[])  [unwired: 2 in, 1 out]
                        n975 = Decimal String To Number(string=w5310) -> (number=w5329:i32[])  [unwired: 2 in, 1 out]
                        n976 = Decimal String To Number(string=w5311) -> (number=w5330:i32[])  [unwired: 2 in, 1 out]
                        n977 = Decimal String To Number(string=w5312) -> (number=w5331:i32[])  [unwired: 2 in, 1 out]
                        n978 = Decimal String To Number(string=w5313) -> (number=w5326:i32[])  [unwired: 2 in, 1 out]
                        n979 = Compound Arithmetic op=ADD(w5303, w5301, w5299, w5297, w5295) -> (w5306:dbl[])
                        n980 = Build Array(w5304) -> (w5325:string[][])
                        n981 = Build Array(w5302) -> (w5324:string[][])
                        n982 = Build Array(w5300) -> (w5323:string[][])
                        n983 = Build Array(w5298) -> (w5322:string[][])
                        n984 = Build Array(w5296) -> (w5321:string[][])
                        n985 = Number To Fractional String(number=w5306, precision (6)=i16 2) -> (F-format string=w5305:string[])  [unwired: 2 in]
                        n986 = Compound Arithmetic op=ADD(w5328, w5329, w5330, w5331, w5326) -> (w5332:i32[])
                        n987 = Transpose 2D Array(2D array=w5325) -> (transposed array=w5319:string[][])
                        n988 = Transpose 2D Array(2D array=w5324) -> (transposed array=w5318:string[][])
                        n989 = Transpose 2D Array(2D array=w5323) -> (transposed array=w5317:string[][])
                        n990 = Transpose 2D Array(2D array=w5322) -> (transposed array=w5316:string[][])
                        n991 = Transpose 2D Array(2D array=w5321) -> (transposed array=w5315:string[][])
                        n992 = Number To Decimal String(number=w5332) -> (decimal integer string=w5327:string[])  [unwired: 1 in]
                        n993 = Build Array(w5305) -> (w5308:string[][])
                        n994 = Transpose 2D Array(2D array=w5308) -> (transposed array=w5314:string[][])
                      }
                      frame #7 {
                        w5336 = string[] [""]
                        n995 = Insert Into Array(array=w5345, index (col)=1 ("disabled index (col)"), new element #1=w5336, new element #2=w5336, new element #3=w5336, new element #4=w5336, new element #5=w5335, new element #6=w5337, new element #7=w5336, new element #8=w5336, new element #9=w5336, new element #10=w5336, new element #11=w5338, new element #12=w5339) -> (w5341:string[][])  [unwired: 1 in]
                        n996 = call "flot graph for month n year.vi"("BD Date"=w5342, "error in (no error)"=w5344, "Count total"=w5338) -> ("error out"=w5343:errorcluster, "Run-Time Status"=w5340:cluster{"Array 2":timestamp[], dbl[]})  [unwired: 7 in]
                        n997 = local write "Run-Time Status"(w5340) -> ()
                        n998 = local write "Table"(w5341) -> ()
                      }
                    }
                  }
                  frame "2" {
                    n999 = flat-sequence {
                      tunnel: w5356 -> [w5470]
                      tunnel: w5355 -> [w5468]
                      tunnel: [w5454] -> w5446
                      tunnel: [w5469] -> w5445
                      tunnel: w5354 -> [_]
                      tunnel: [w5473] -> w5444
                      tunnel: [w5453] -> w5443
                      tunnel: [w5452] -> w5442
                      tunnel: [w5451] -> w5441
                      tunnel: w5353 -> [w5453]
                      tunnel: w5352 -> [w5452]
                      tunnel: ["Where BREAKDOWN_DATE between '%s'and '%s' and BREAKDOWN_STK_HOLD_ID ='%d' and  SHIFT_ID = '%d' "] -> w5440
                      tunnel: [w5451] -> w5439
                      tunnel: w5351 -> [w5447]
                      tunnel: [w5447] -> w5350
                      tunnel: w5446 -> [w5534]
                      tunnel: w5445 -> [w5536]
                      tunnel: w5444 -> [w5532]
                      tunnel: w5443 -> [w5531]
                      tunnel: w5442 -> [w5530]
                      tunnel: [w5533] -> w5438
                      tunnel: [w5535] -> w5437
                      tunnel: [w5532] -> w5436
                      tunnel: [w5522] -> w5435
                      tunnel: [w5528] -> w5434
                      tunnel: [w5531] -> w5433
                      tunnel: [w5530] -> w5432
                      tunnel: w5441 -> [w5527]
                      tunnel: [w5527] -> w5431
                      tunnel: w5440 -> [w5524]
                      tunnel: [w5524] -> w5430
                      tunnel: [w5523] -> w5429
                      tunnel: w5439 -> [w5523]
                      tunnel: w5350 -> [w5521]
                      tunnel: [w5520] -> w5349
                      tunnel: w5438 -> [w5566]
                      tunnel: w5437 -> [w5564]
                      tunnel: w5436 -> [w5569]
                      tunnel: w5435 -> [w5568]
                      tunnel: w5434 -> [w5567]
                      tunnel: w5433 -> [w5562]
                      tunnel: w5432 -> [w5561]
                      tunnel: [w5569] -> w5428
                      tunnel: [w5568] -> w5427
                      tunnel: [w5567] -> w5426
                      tunnel: [w5565] -> w5425
                      tunnel: [w5559] -> w5424
                      tunnel: [w5558] -> w5423
                      tunnel: [w5563] -> w5422
                      tunnel: [w5562] -> w5421
                      tunnel: [w5561] -> w5420
                      tunnel: w5431 -> [w5557]
                      tunnel: [w5557] -> w5419
                      tunnel: w5430 -> [w5554]
                      tunnel: [w5554] -> w5418
                      tunnel: [w5553] -> w5417
                      tunnel: w5429 -> [w5553]
                      tunnel: w5349 -> [w5552]
                      tunnel: [w5551] -> w5348
                      tunnel: w5428 -> [w5604]
                      tunnel: w5427 -> [w5603]
                      tunnel: w5426 -> [w5602]
                      tunnel: w5425 -> [w5599]
                      tunnel: w5424 -> [w5601]
                      tunnel: w5423 -> [w5600]
                      tunnel: w5422 -> [w5597]
                      tunnel: w5421 -> [w5595]
                      tunnel: w5420 -> [w5594]
                      tunnel: [w5604] -> w5416
                      tunnel: [w5603] -> w5415
                      tunnel: [w5602] -> w5414
                      tunnel: [w5601] -> w5413
                      tunnel: [w5600] -> w5412
                      tunnel: [w5598] -> w5411
                      tunnel: [w5592] -> w5410
                      tunnel: [w5591] -> w5409
                      tunnel: [w5596] -> w5408
                      tunnel: [w5595] -> w5407
                      tunnel: [w5594] -> w5406
                      tunnel: w5419 -> [w5590]
                      tunnel: [w5590] -> w5405
                      tunnel: w5418 -> [w5587]
                      tunnel: [w5587] -> w5404
                      tunnel: [w5586] -> w5403
                      tunnel: w5417 -> [w5586]
                      tunnel: w5348 -> [w5584]
                      tunnel: w5416 -> [w5625]
                      tunnel: w5415 -> [w5624]
                      tunnel: w5414 -> [w5623]
                      tunnel: w5413 -> [w5622]
                      tunnel: w5412 -> [w5621]
                      tunnel: w5411 -> [w5618]
                      tunnel: w5410 -> [w5620]
                      tunnel: w5409 -> [w5619]
                      tunnel: w5408 -> [w5617]
                      tunnel: w5407 -> [w5614]
                      tunnel: w5406 -> [w5613]
                      tunnel: [w5625] -> w5402
                      tunnel: [w5624] -> w5401
                      tunnel: [w5623] -> w5400
                      tunnel: [w5622] -> w5399
                      tunnel: [w5621] -> w5398
                      tunnel: [w5620] -> w5397
                      tunnel: [w5619] -> w5396
                      tunnel: [w5616] -> w5395
                      tunnel: [w5615] -> w5394
                      tunnel: [w5611] -> w5393
                      tunnel: [w5610] -> w5392
                      tunnel: [w5614] -> w5391
                      tunnel: [w5613] -> w5390
                      tunnel: w5405 -> [w5609]
                      tunnel: [w5609] -> w5389
                      tunnel: w5404 -> [w5606]
                      tunnel: [w5606] -> w5388
                      tunnel: [w5605] -> w5387
                      tunnel: w5403 -> [w5605]
                      tunnel: w5402 -> [w5660]
                      tunnel: w5401 -> [w5659]
                      tunnel: w5400 -> [w5658]
                      tunnel: w5399 -> [w5657]
                      tunnel: w5398 -> [w5656]
                      tunnel: w5397 -> [w5655]
                      tunnel: w5396 -> [w5654]
                      tunnel: w5395 -> [w5649]
                      tunnel: w5394 -> [w5651]
                      tunnel: w5393 -> [w5653]
                      tunnel: w5392 -> [w5652]
                      tunnel: w5391 -> [w5646]
                      tunnel: w5390 -> [w5647]
                      tunnel: [w5660] -> w5386
                      tunnel: [w5659] -> w5385
                      tunnel: [w5658] -> w5384
                      tunnel: [w5657] -> w5383
                      tunnel: [w5656] -> w5382
                      tunnel: [w5655] -> w5381
                      tunnel: [w5654] -> w5380
                      tunnel: [w5653] -> w5379
                      tunnel: [w5652] -> w5378
                      tunnel: [w5650] -> w5377
                      tunnel: [w5648] -> w5376
                      tunnel: [w5644] -> w5375
                      tunnel: [w5642] -> w5374
                      tunnel: w5389 -> [w5643]
                      tunnel: w5388 -> [w5639]
                      tunnel: [w5638] -> w5373
                      tunnel: w5387 -> [w5638]
                      tunnel: w5386 -> [w5699]
                      tunnel: w5385 -> [w5692]
                      tunnel: w5384 -> [w5683]
                      tunnel: w5383 -> [w5691]
                      tunnel: w5382 -> [w5681]
                      tunnel: w5381 -> [w5690]
                      tunnel: w5380 -> [w5679]
                      tunnel: w5379 -> [w5689]
                      tunnel: w5378 -> [w5677]
                      tunnel: w5377 -> [w5713]
                      tunnel: w5376 -> [w5712]
                      tunnel: w5375 -> [w5688]
                      tunnel: w5374 -> [w5675]
                      tunnel: [w5713] -> w5372
                      tunnel: [w5712] -> w5371
                      tunnel: [w5706] -> w5370
                      tunnel: [w5699] -> w5369
                      tunnel: [w5698] -> w5368
                      tunnel: [w5697] -> w5367
                      tunnel: [w5696] -> w5366
                      tunnel: [w5695] -> w5365
                      tunnel: [w5694] -> w5364
                      tunnel: [w5693] -> w5363
                      tunnel: [w5692] -> w5362
                      tunnel: [w5691] -> w5361
                      tunnel: [w5690] -> w5360
                      tunnel: [w5689] -> w5359
                      tunnel: [w5688] -> w5358
                      tunnel: [w5673] -> w5357
                      tunnel: w5373 -> [w5673]
                      tunnel: [w5726] -> _
                      tunnel: [w5722] -> _
                      tunnel: w5372 -> [w5723]
                      tunnel: w5371 -> [w5726]
                      tunnel: w5370 -> [w5717]
                      tunnel: w5369 -> [w5724]
                      tunnel: w5368 -> [_]
                      tunnel: w5367 -> [_]
                      tunnel: w5366 -> [w5716]
                      tunnel: w5365 -> [_]
                      tunnel: w5364 -> [_]
                      tunnel: w5363 -> [w5718]
                      tunnel: w5362 -> [_]
                      tunnel: w5361 -> [_]
                      tunnel: w5360 -> [w5714]
                      tunnel: w5359 -> [_]
                      tunnel: w5358 -> [_]
                      tunnel: w5357 -> [w5721]
                      frame #0 {
                        w5461 = "%Y-%m-%d" ("time format string (%c)")
                        n1000 = Decimal String To Number(string=w5447) -> (number=w5448:i32)  [unwired: 2 in, 1 out]
                        n1001 = property on="Table" class="Tbl (strict)"("Visible"=TRUE) -> ()  [unwired: 2 in, 2 out]
                        n1002 = Format Date/Time String(time format string (%c)=w5461, seconds (now)=w5453) -> (date/time string=w5462:string)  [unwired: 1 in]
                        n1003 = Format Date/Time String(time format string (%c)=w5461, seconds (now)=w5452) -> (date/time string=w5460:string)  [unwired: 1 in]
                        n1004 = Format Into String(format string="Where BREAKDOWN_DATE between '%s' and '%s' and  SHIFT_ID = '%d'  ", w5462, w5460, w5448) -> (resulting string=w5459:string)  [unwired: 2 in, 1 out]
                        n1005 = call <vilib>:"DB Tools Select Data.vi"("condition"=w5459, "error in (no error)"=w5468, "columns"=string[] ["BREAKDOWN_DATE"], "table"="STATION_1_LOG_HISTORY", "connection reference"=w5470) -> ("error out"=w5455:errorcluster, "data"=w5458:variant[][], "connection reference out"=w5469:T2)  [unwired: 1 in]
                        n1006 = property on="Table 2" class="Tbl (strict)"("Visible"=FALSE) -> ()  [unwired: 2 in, 2 out]
                        n1007 = xnode "Database Variant To Data"("database variant"=w5458, "error in (no error)"=w5455, "type"=string[][] [] ("Elements Found")) -> ("data"=w5456:string[][], "error out"=w5454:errorcluster)
                        n1008 = Index Array(array=w5456, index (col)=0 ("disabled index (col)")) -> (element=w5464:string[])  [unwired: 1 in]
                        n1009 = call "Search_1d_array_element.vi"("Count in"=string[] [] ("Elements Found"), "BD Date"=w5464, "Elements Found in"=string[] [] ("Elements Found")) -> ("Elements Found out"=w5451:string[])  [unwired: 4 in, 2 out]
                        n1010 = Build Array(w5451) -> (w5474:string[][])
                        n1011 = Transpose 2D Array(2D array=w5474) -> (transposed array=w5473:string[][])
                      }
                      frame #1 {
                        n1012 = disable-structure shown="Enabled" {
                          disable-tunnel: w5536 -> [w5547 w5549]
                          disable-tunnel: [w5546 w5549] -> w5535
                          disable-tunnel: w5534 -> [w5545 w5550]
                          disable-tunnel: [w5544 w5550] -> w5533
                          disable-tunnel: w5531 -> [w5542 _]
                          disable-tunnel: w5530 -> [w5541 _]
                          disable-tunnel: [w5540 _] -> w5529
                          disable-tunnel: [w5539 _] -> w5526
                          disable-tunnel: w5524 -> [w5538 _]
                          disable-tunnel: w5521 -> [w5537 w5548]
                          disable-tunnel: [_ w5548] -> w5520
                          frame Disabled {
                            n1013 = call "Stack_holderwise_total_bd_count_&_duration_2.vi"("Refnum in"=w5547, "BREAKDOWN_STK_HOLD_ID"=1, "condition"=w5538, "Form Date"=w5542, "To Date"=w5541, "error in (no error)"=w5545, "Shift"=w5537) -> ("Refnum out"=w5546:T2, "Count out"=w5540:string[], "appended array"=w5539:dbl[], "error out"=w5544:errorcluster)  [unwired: 5 in]
                          }
                          frame Enabled {
                          }
                        }
                        n1014 = call "NUMERIC TO STRING.vi"("appended array"=w5526) -> ("Array"=w5525:string[])  [unwired: 4 in]
                        n1015 = call "Insert_empty_element_with_zero.vi"("searched date"=w5529, "fixed date"=w5527) -> ("O/P"=w5522:string[])  [unwired: 9 in]
                        n1016 = call "Insert_empty_element_with_zero.vi"("searched date"=w5525, "fixed date"=w5527) -> ("O/P"=w5528:string[])  [unwired: 9 in]
                      }
                      frame #2 {
                        n1017 = disable-structure shown="Enabled" {
                          disable-tunnel: w5566 -> [w5580 w5582]
                          disable-tunnel: [w5579 w5582] -> w5565
                          disable-tunnel: w5564 -> [w5578 w5583]
                          disable-tunnel: [w5577 w5583] -> w5563
                          disable-tunnel: w5562 -> [w5576 _]
                          disable-tunnel: w5561 -> [w5575 _]
                          disable-tunnel: [w5574 _] -> w5560
                          disable-tunnel: [w5573 _] -> w5556
                          disable-tunnel: w5554 -> [w5572 _]
                          disable-tunnel: w5552 -> [w5570 w5581]
                          disable-tunnel: [_ w5581] -> w5551
                          frame Disabled {
                            n1018 = call "Stack_holderwise_total_bd_count_&_duration_2.vi"("Refnum in"=w5578, "BREAKDOWN_STK_HOLD_ID"=2, "condition"=w5572, "Form Date"=w5576, "To Date"=w5575, "error in (no error)"=w5580, "Shift"=w5570) -> ("Refnum out"=w5577:T2, "Count out"=w5574:string[], "appended array"=w5573:dbl[], "error out"=w5579:errorcluster)  [unwired: 5 in]
                          }
                          frame Enabled {
                          }
                        }
                        n1019 = call "Insert_empty_element_with_zero.vi"("searched date"=w5560, "fixed date"=w5557) -> ("O/P"=w5559:string[])  [unwired: 9 in]
                        n1020 = call "NUMERIC TO STRING.vi"("appended array"=w5556) -> ("Array"=w5555:string[])  [unwired: 4 in]
                        n1021 = call "Insert_empty_element_with_zero.vi"("searched date"=w5555, "fixed date"=w5557) -> ("O/P"=w5558:string[])  [unwired: 9 in]
                      }
                      frame #3 {
                        n1022 = call "Stack_holderwise_total_bd_count_&_duration_2.vi"("Refnum in"=w5597, "BREAKDOWN_STK_HOLD_ID"=3, "condition"=w5587, "Form Date"=w5595, "To Date"=w5594, "error in (no error)"=w5599, "Shift"=w5584) -> ("Refnum out"=w5596:T2, "Count out"=w5593:string[], "appended array"=w5589:dbl[], "error out"=w5598:errorcluster)  [unwired: 5 in]
                        n1023 = call "Insert_empty_element_with_zero.vi"("searched date"=w5593, "fixed date"=w5590) -> ("O/P"=w5592:string[])  [unwired: 9 in]
                        n1024 = call "NUMERIC TO STRING.vi"("appended array"=w5589) -> ("Array"=w5588:string[])  [unwired: 4 in]
                        n1025 = call "Insert_empty_element_with_zero.vi"("searched date"=w5588, "fixed date"=w5590) -> ("O/P"=w5591:string[])  [unwired: 9 in]
                      }
                      frame #4 {
                        n1026 = disable-structure shown="Enabled" {
                          disable-tunnel: w5618 -> [w5634 w5637]
                          disable-tunnel: w5617 -> [w5633 w5636]
                          disable-tunnel: [w5632 w5636] -> w5616
                          disable-tunnel: [w5631 w5637] -> w5615
                          disable-tunnel: w5614 -> [w5630 _]
                          disable-tunnel: w5613 -> [w5629 _]
                          disable-tunnel: [w5628 _] -> w5612
                          disable-tunnel: [w5627 _] -> w5608
                          disable-tunnel: w5606 -> [w5626 _]
                          frame Disabled {
                            n1027 = call "Stack_holderwise_total_bd_count_&_duration.vi"("Refnum in"=w5633, "BREAKDOWN_STK_HOLD_ID"=4, "condition"=w5626, "Form Date"=w5630, "To Date"=w5629, "error in (no error)"=w5634) -> ("Refnum out"=w5632:T2, "Count out"=w5628:string[], "appended array"=w5627:dbl[], "error out"=w5631:errorcluster)  [unwired: 6 in]
                          }
                          frame Enabled {
                          }
                        }
                        n1028 = call "Insert_empty_element_with_zero.vi"("searched date"=w5612, "fixed date"=w5609) -> ("O/P"=w5611:string[])  [unwired: 9 in]
                        n1029 = call "NUMERIC TO STRING.vi"("appended array"=w5608) -> ("Array"=w5607:string[])  [unwired: 4 in]
                        n1030 = call "Insert_empty_element_with_zero.vi"("searched date"=w5607, "fixed date"=w5609) -> ("O/P"=w5610:string[])  [unwired: 9 in]
                      }
                      frame #5 {
                        n1031 = disable-structure shown="Enabled" {
                          disable-tunnel: w5651 -> [w5669 w5672]
                          disable-tunnel: [w5668 w5672] -> w5650
                          disable-tunnel: w5649 -> [w5667 w5671]
                          disable-tunnel: [w5666 w5671] -> w5648
                          disable-tunnel: w5647 -> [w5665 _]
                          disable-tunnel: w5646 -> [w5664 _]
                          disable-tunnel: [w5663 _] -> w5645
                          disable-tunnel: [w5662 _] -> w5641
                          disable-tunnel: w5639 -> [w5661 _]
                          frame Disabled {
